vi "0037-Sub_CP2112_SHT31_2.vi"(8 "エラー入力（エラーなし）":errorcluster, 10 "slaveAddress":u8, 11 "device":T1) -> (0 "エラー出力":errorcluster, 2 "相対湿度":dbl, 3 "温度":dbl)   [LabVIEW 2014]
uses:
  LVProject/private/CP2112_device.ctl
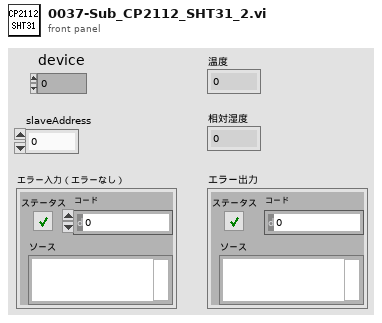
[diagram p1: front panel]
types:
  T1 = typedef "CP2112_device.ctl" = i32
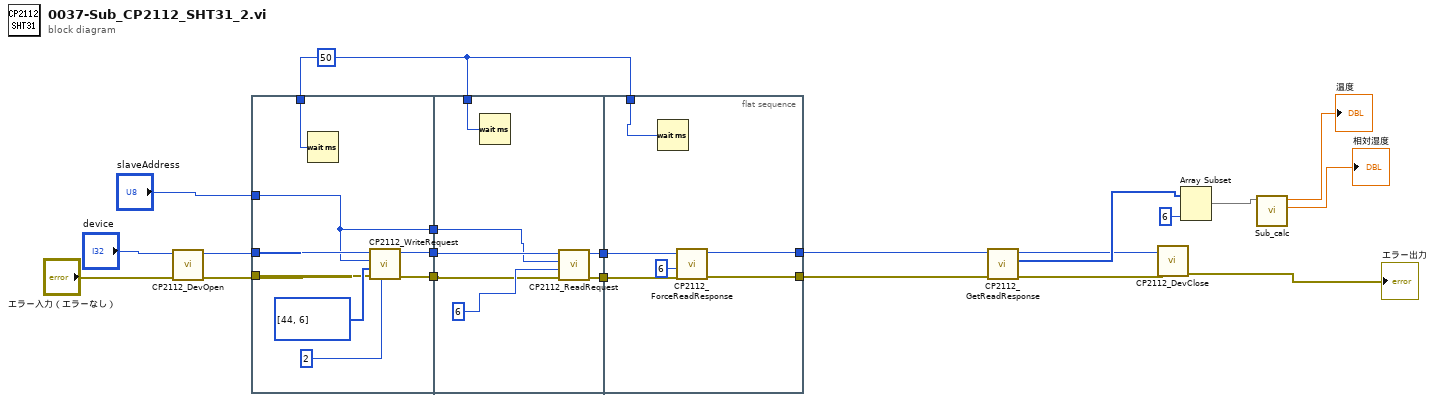
[diagram p0: block diagram]
diagram:
  w14 = u32 50 ("ミリ秒待機時間")
  n1 = call "CP2112_DevOpen.vi"("error in (no error)"="エラー入力（エラーなし）", "deviceNum"="device") -> ("error out"=w6:errorcluster, "device"=w5:T1)  [unwired: 7 in, 1 out]
  n2 = flat-sequence {
    tunnel: [w25] -> w21
    tunnel: [w24] -> w20
    tunnel: w14 -> [w23]
    tunnel: w5 -> [w27]
    tunnel: w6 -> [w26]
    tunnel: "slaveAddress" -> [w22]
    tunnel: [w22] -> w19
    tunnel: w21 -> [w34]
    tunnel: w20 -> [w35]
    tunnel: [w33] -> w18
    tunnel: [w32] -> w17
    tunnel: w14 -> [w31]
    tunnel: w19 -> [w30]
    tunnel: w18 -> [w41]
    tunnel: w17 -> [w40]
    tunnel: [w39] -> w7
    tunnel: [w38] -> w8
    tunnel: w14 -> [w37]
    frame #0 {
      n3 = Wait (ms)(milliseconds to wait=w23) -> ()  [unwired: 1 out]
      n4 = call "CP2112_WriteRequest.vi"("numBytesToWrite"=i16 2 ("numByteToRead"), "error in (no error)"=w26, "buffer"=u8[] [44, 6], "slaveAddress"=w22, "device"=w27) -> ("error out"=w25:errorcluster, "deviceOut"=w24:T1)  [unwired: 4 in, 1 out]
    }
    frame #1 {
      n5 = Wait (ms)(milliseconds to wait=w31) -> ()  [unwired: 1 out]
      n6 = call "CP2112_ReadRequest.vi"("error in (no error)"=w34, "numByteToRead"=i16 6, "slaveAddress"=w30, "device"=w35) -> ("error out"=w32:errorcluster, "deviceOut"=w33:T1)  [unwired: 5 in, 1 out]
    }
    frame #2 {
      n7 = Wait (ms)(milliseconds to wait=w37) -> ()  [unwired: 1 out]
      n8 = call "CP2112_ForceReadResponse.vi"("error in (no error)"=w40, "numByteToRead"=i16 6, "device"=w41) -> ("error out"=w38:errorcluster, "deviceOut"=w39:T1)  [unwired: 6 in, 1 out]
    }
  }
  n9 = call "CP2112_GetReadResponse.vi"("error in (no error)"=w8, "device"=w7) -> ("error out"=w4:errorcluster, "buffer"=w10:u8[], "deviceOut"=w3:T1)  [unwired: 4 in, 3 out]
  n10 = call "CP2112_DevClose.vi"("error in (no error)"=w4, "device"=w3) -> ("error out"=→"エラー出力":errorcluster)  [unwired: 9 in]
  n11 = Array Subset(array=w10, length=6 ("長さ")) -> (w11:u8[])  [unwired: 1 in]
  n12 = call "Sub_calc.vi"("Data"=w11) -> ("数値"=→"相対湿度":dbl, "数値 2"=→"温度":dbl)  [unwired: 9 in]
